vi "TCP Error Handler.vi"(8 "Error In":errorcluster, 11 "TCP State In":T1) -> (0 "error out":errorcluster, 3 "TCP State Out":T1)   [LabVIEW 2019]
uses:
  TCP send commands.ctl
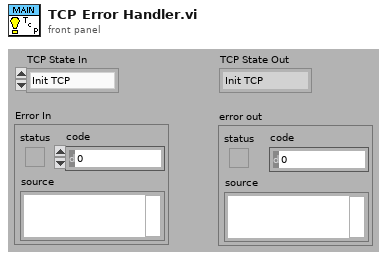
[diagram p1: front panel]
types:
  T1 = typedef "TCP send commands.ctl" = enum16{"Init TCP", "Close TCP & Stop", "TCP Connected", "Close TCP & Init"}
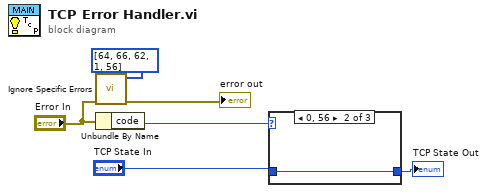
[diagram p0: block diagram]
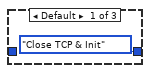
[diagram p2: hidden frame]
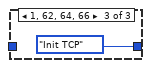
[diagram p3: hidden frame]
diagram:
  n1 = call "Ignore Specific Errors.vi"("error in (no error)"="Error In", "Array"=i32[] [64, 66, 62, 1, 56]) -> ("error out"=→"error out":errorcluster)  [unwired: 8 in, 1 out]
  n2 = Unbundle By Name("Error In") -> ("code"=w6:i32)
  n3 = case shown="0, 56" w6 {
    tunnel: [TCP_send_commands."Close TCP & Init" ("Enum") w8 TCP_send_commands."Init TCP" ("Enum")] -> w4
    tunnel: "TCP State In" -> [_ w8 _]
    frame Default {
    }
    frame 0, 56 {
    }
    frame 1, 62, 64, 66 {
    }
  }
  "TCP State Out" <- w4
